vi "10-send&receive-arrays-backup2.vi"() -> ()   [LabVIEW 2018]
uses:
  LV2Julia_core/VIs/Server or client state.ctl
  LV2Julia_core/VIs/detailed error info.ctl
  LV2Julia_core/VIs/StackFrame.ctl
  LV2Julia_core/VIs/Numeric Types enum.ctl
  array 123D sizes.ctl
  LV2Julia_core/VIs/Commands.ctl
  19565153-6e23-41a7-814d-e58de81dde5a.vi
  5ef99b4f-9bfc-4a0d-a8a0-74b261859f3d.vi
  388a3b2a-e541-4e37-ba3b-5749cefc77c1.vi
  e91abbe1-2489-4f0d-9743-379a6a4cbf4d.vi
  19565153-6e23-41a7-814d-e58de81dde5a.vi/85887d54-d509-450b-84bb-3c420582994f.vi
  <vilib>/Utility/High Resolution Relative Seconds.vi
  388a3b2a-e541-4e37-ba3b-5749cefc77c1.vi/1b30b06e-7fd1-4fdb-a624-ecc8bbac65c1.vi
  19565153-6e23-41a7-814d-e58de81dde5a.vi/85887d54-d509-450b-84bb-3c420582994f.vi/d3e8bd18-7aca-49eb-9cc1-8936944af3d1.vi
  19565153-6e23-41a7-814d-e58de81dde5a.vi/85887d54-d509-450b-84bb-3c420582994f.vi/cc0638ed-03b9-4f11-90bc-5f951413100e.vi
  19565153-6e23-41a7-814d-e58de81dde5a.vi/85887d54-d509-450b-84bb-3c420582994f.vi/437cd6de-f34e-42af-877a-dd33a1fabbe3.vi
  388a3b2a-e541-4e37-ba3b-5749cefc77c1.vi/1b30b06e-7fd1-4fdb-a624-ecc8bbac65c1.vi/cb39e787-6450-4332-a618-a02e848b2eda.vi
  388a3b2a-e541-4e37-ba3b-5749cefc77c1.vi/1b30b06e-7fd1-4fdb-a624-ecc8bbac65c1.vi/8ffec59d-6774-4d31-b6e2-7d50134dbb1f.vi
  388a3b2a-e541-4e37-ba3b-5749cefc77c1.vi/1b30b06e-7fd1-4fdb-a624-ecc8bbac65c1.vi/38fcd616-394b-4d55-b8d7-64853e38e30b.vi
  LV2Julia_core/VIs/jl-scripts path.vi
  LV2Julia_core/VIs/check ID validity.vi
  LV2Julia_core/VIs/bindata_descr to JSON.vi
  LV2Julia_core/VIs/check cluster field names.vi
  LV2Julia_core/VIs/concat JSON.vi
  LV2Julia_core/VIs/build request.vi
  LV2Julia_core/VIs/Parse server response.vi
  LV2Julia_core/VIs/log jl exceptions.vi
  LV2Julia_core/LV2Julia_core.lvlib
  LV2Julia_examples.lvlib
panel:
  out "ZMQ timeout":bool
  out "Julia script file path":path
  out "temporary script path":path
  in  "execution control pages":enum32{"Start&stop", "go - test", "error"}(tab)
  in  "returnarrs":bool=TRUE
  in  "go":bool caption="go (Julia Server started externally)"
  in  "Start with Julia":bool caption="Start Julia Server and go"
  in  "ZMQ endpoint":string="tcp://127.0.0.1:5555"
  out "Jl Server state":T1
  in  "stop this VI only":bool
  in  "stop both this VI and Julia Server":bool
  in  "Stop JL-server":bool
  in  "log2(arrsize)":u32=7 min=5
  in  "cycle min time (s)":sgl min=0 step=0.2
  out "numarray 3D":cdb[][][](array[numeric])
  out "numarray 2D":cdb[][](array[numeric])
  out "numarray 1D":cdb[](array[numeric]) format="%.1f"
  out "numeric type":T2
  out "arr dimension":i32
  out "all arrays OK":bool
  out "arrs equal":bool
  out "array sizes":T3
  out "el_type":string
  out "arsize":i32[](array[numeric])
  out "data flattening delta t":dbl
  out "flattening ms/MB":dbl format="%#.2f"
  out "Zmq&Julia delta t":dbl
  out "Zmq&JUlia ms/MB":dbl format="%#.2f"
  out "data unflattening delta t":dbl
  out "unflattening ms/MB":dbl format="%#.2f"
  out "detailed error info":T4
  out "current error":errorcluster
  out "final error":errorcluster
  out "short err code":u8
  # "tcp://127.0.0.1:5555 \nfor local Julia Server\n\nFor a Julia Server running on a separate computer,  you probably must use an IPv4 address in numeric form (not a DNS name) - see https://stackoverflow.com/questions/6024003/why-doesnt-zeromq-work-on-localhost.\n\nFor instructions how to properly start the corresponding Julia script, see \n05-on_external_server.jl file in the jl-scripts folder.\n\nThe ZMQ endpoint control only used if Julia Server is not being started by this VI."
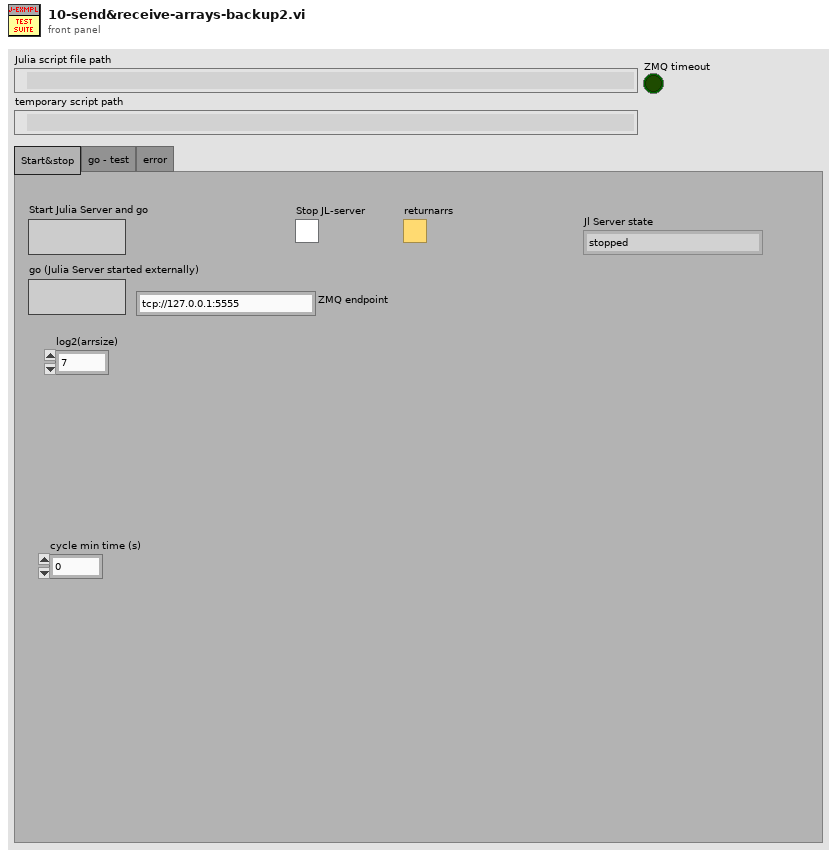
[diagram p1: front panel]
types:
  T1 = typedef "LV2Julia_core.lvlib/Server or client state.ctl" = enum16{"stopped", "running", "unknown"}
  T2 = typedef "LV2Julia_core.lvlib/Numeric Types enum.ctl" = enum16{"SGL", "DBL", "I8", "I16", "I32", "I64", "U8", "U16", "U32", "U64", "CSGL", "CDBL", "boolean"}
  T3 = typedef "array 123D sizes.ctl" = cluster{"s1":i32, "s2":i32[], "s3":i32[]}
  T4 = typedef "LV2Julia_core.lvlib/detailed error info.ctl" = cluster{"exception_or_info":string, "trace":T5[]}
  T5 = typedef "LV2Julia_core.lvlib/StackFrame.ctl" = cluster{"frame_summary":string, "func":string, "linfo":string, "file":string, "line":i32, "pointer":u64, "from_c":bool, "inlined":bool}
  T6 = typedef "LV2Julia_core.lvlib/Commands.ctl" = enum16{"Start Jl-server & Init LV-client", "Send request & Get response ", "Stop Jl-server & Cleanup LV-client", "Cleanup LV-client", "Start Jl-server", "Stop Jl-server", "Init LV-Client", "Cleanup LV-Client", "(not allowed)", "Set LV Client state", "Set Jl Server state", "set ZMQ timeout", "read ZMQ timeout", "read-out state"}
  T7 = typedef "LV2Julia_core.lvlib/Bindata&description.ctl" = cluster{"bindata_descr":T8[], "bindata":u8[]}
  T8 = typedef "LV2Julia_core.lvlib/Bindata description.ctl" = cluster{"nofbytes":i32, "numtype":string, "start":i32, "arrdims":i32[], "kwarg_name":string, "category":string}
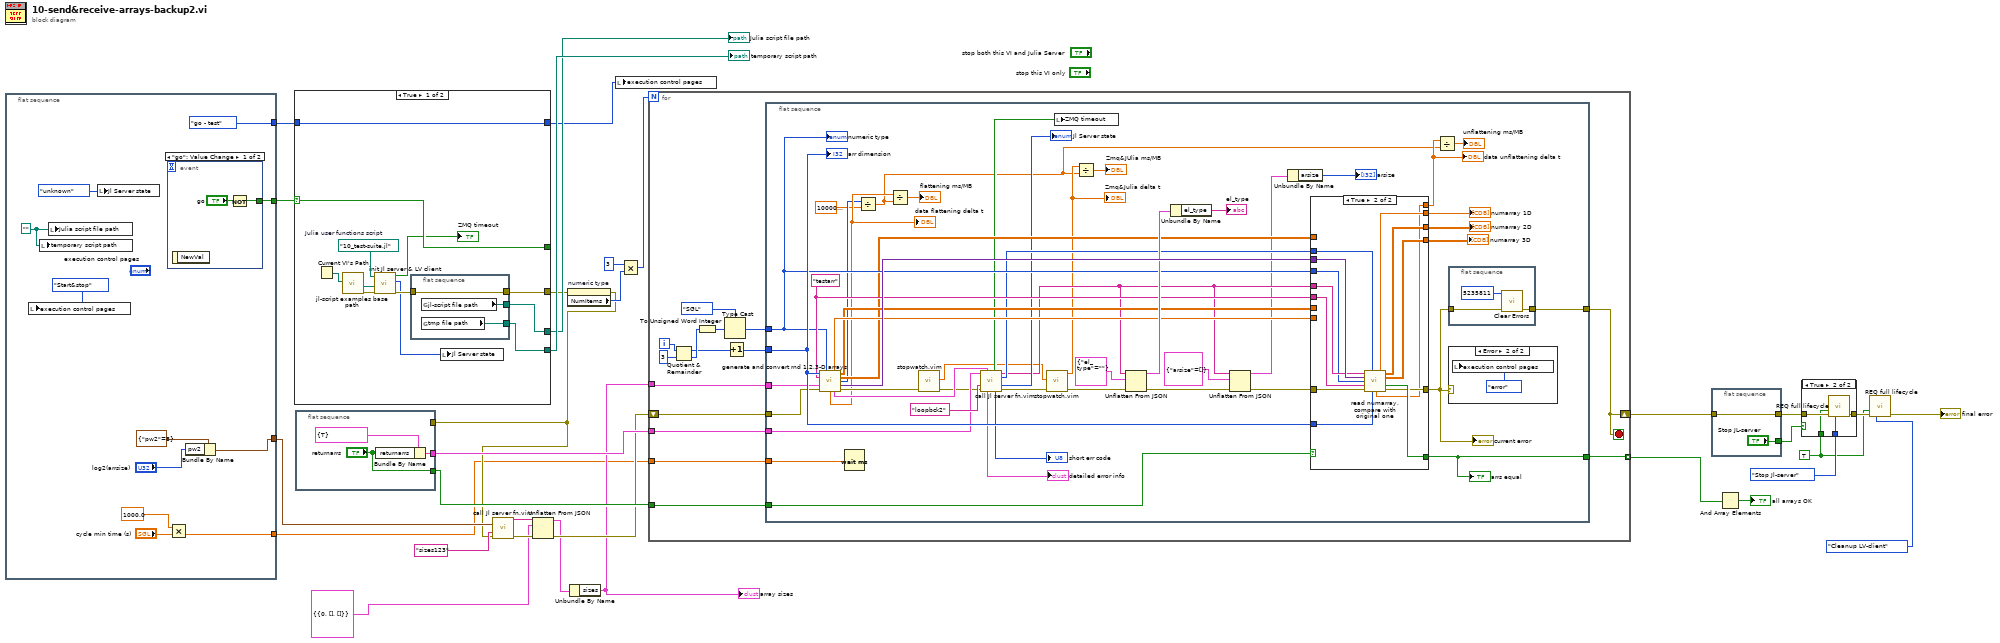
[diagram p0: block diagram]
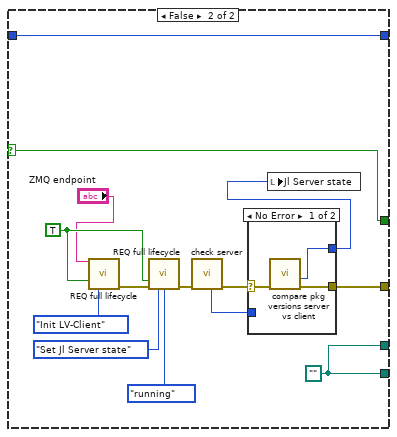
[diagram p2: hidden frame]
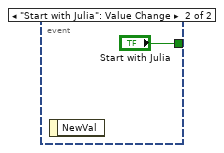
[diagram p4: hidden frame]
diagram:
  w27 = TRUE ("Force command")
  n1 = flat-sequence {
    tunnel: [w40] -> w20
    tunnel: [enum32{"Start&stop", "go - test", "error"}."go - test" ("execution control pages")] -> w15
    tunnel: [w36] -> w9
    tunnel: [w33] -> w1
    frame #0 {
      w41 = path ""
      n2 = local write "execution control pages"(enum32{"Start&stop", "go - test", "error"}."Start&stop" ("execution control pages")) -> ()
      n3 = local write "temporary script path"(w41) -> ()
      n4 = local write "Julia script file path"(w41) -> ()
      n5 = local write "Jl Server state"(Server_or_client_state."unknown" ("Jl Server state out")) -> ()
      n6 = event shown="[0] \"go\": Value Change" {
        selector: _ -> [_ _]
        dyn-events: _ -> [_ _]
        timeout: _ -> [_ _]
        tunnel: [w43 "Start with Julia"] -> w40
        event "go": Value Change {
          n7 = event-data() -> ()  [unwired: 1 in, 1 out]
          n8 = Not(x="go") -> (.not. x?=w43:bool)
        }
        event "Start with Julia": Value Change {
          n9 = event-data() -> ()  [unwired: 1 in, 1 out]
        }
      }
      n10 = Multiply(x=sgl 1000.0, y="cycle min time (s)") -> (x*y=w33:sgl)
      n11 = Bundle By Name(cluster=cluster{"pw2":u32} {"pw2"=8}, "pw2"="log2(arrsize)") -> (w36:cluster{"pw2":u32})
    }
  }
  n12 = case shown="True" w20 {
    selector: w20 -> [w57 w70]
    tunnel: [w56 w65] -> w17
    tunnel: [w57 w70] -> _
    tunnel: [w55 w67] -> w18
    tunnel: [w54 w67] -> w19
    tunnel: [w46 w61] -> w16
    tunnel: w15 -> [w46 w61]
    frame True {
      w48 = path "10_test-suite.jl"  # Julia user functions script
      n13 = Current VI's Path() -> (path=w52:path)
      n14 = call "jl-script examples base path.vi"("calling example VI path"=w52) -> ("error out"=w51:errorcluster, "jl-script-examples base path"=w50:path)  [unwired: 9 in]
      n15 = call "init Jl server & LV client.vi"("error in (no error)"=w51, "Base path (not a path)"=w50, "Julia user functions script"=w48) -> ("error out"=w53:errorcluster, "Jl Server state out"=w49:T1, "timeout?"=→"ZMQ timeout":bool)  [unwired: 6 in]
      n16 = flat-sequence {
        tunnel: [w60] -> w56
        tunnel: w53 -> [w60]
        tunnel: [w59] -> w55
        tunnel: [w58] -> w54
        frame #0 {
          n17 = global read "jl-scripts path.vi" "jl-script file path"() -> (w59:path)
          n18 = global read "jl-scripts path.vi" "tmp file path"() -> (w58:path)
        }
      }
      n19 = local write "Jl Server state"(w49) -> ()
    }
    frame False {
      w67 = path ""
      w72 = TRUE ("Force command")
      n20 = call "REQ full lifecycle.vi"("ZMQ endpoint"="ZMQ endpoint", "Force command"=w72, "command"=Commands."Init LV-Client") -> ("error out"=w69:errorcluster)  [unwired: 6 in, 6 out]
      n21 = call "REQ full lifecycle.vi"("Force command"=w72, "error in"=w69, "command"=Commands."Set Jl Server state", "Jl Server state in"=Server_or_client_state."running") -> ("error out"=w68:errorcluster)  [unwired: 5 in, 6 out]
      n22 = call "check server.vi"("error in"=w68) -> ("error out"=w66:errorcluster, "Jl Server state out"=w64:T1)  [unwired: 6 in, 3 out]
      n23 = case shown="No Error" w66 {
        selector: w66 -> [w77 w79]
        tunnel: [w76 w79] -> w65
        tunnel: [w75 w78] -> w62
        tunnel: w64 -> [_ w78]
        frame No Error {
          n24 = call "compare pkg versions server vs client.vi"("error in (no error)"=w77) -> ("error out"=w76:errorcluster, "Jl Server state out"=w75:T1)  [unwired: 4 in, 5 out]
        }
        frame Error {
        }
      }
      n25 = local write "Jl Server state"(w62) -> ()
    }
  }
  "temporary script path" <- w19
  "Julia script file path" <- w18
  n26 = flat-sequence {
    tunnel: [w81] -> w14
    tunnel: ["returnarrs"] -> w13
    tunnel: w8 -> [_]
    frame #0 {
      n27 = Bundle By Name(cluster=cluster{"returnarrs":bool} {"returnarrs"=TRUE}, "returnarrs"="returnarrs") -> (w81:cluster{"returnarrs":bool})
    }
  }
  n28 = property on="numeric type" class="Enum (strict)"(error in=w17) -> (error out=w8:errorcluster, "NumItems"=w25:u32)  [unwired: 1 in, 1 out]
  n29 = call "call Jl server fn.vim"("Arguments 2"=w9, "fun2call"="sizes123", "error in (no error)"=w8) -> ("JSON received"=w5:string, "error out"=w7:errorcluster)  [unwired: 6 in, 5 out]
  n30 = Unflatten From JSON(JSON string=w5, type and defaults=cluster{"sizes":T3} {"sizes"={"s1"=0, "s2"=[], "s3"=[]}}, error in (no error)=w7) -> (value=w4:cluster{"sizes":T3}, error out=w6:errorcluster)  [unwired: 4 in]
  n31 = Unbundle By Name(w4) -> ("sizes"=w2:T3)
  "array sizes" <- w2
  n32 = local write "execution control pages"(w16) -> ()
  n33 = Multiply(x=u32 3, y=w25) -> (x*y=w23:u32)
  n34 = for {
    N: w23 -> [_]
    tunnel: [w83] -> w22 mode=indexing
    shift-right: [w89] -> w12
    shift-left: w6 -> [w90]
    tunnel: w14 -> [w86]
    tunnel: w13 -> [w87]
    tunnel: w2 -> [w85]
    tunnel: w1 -> [w84]
    i -> [w97]
    stop <- w89 stop-if-true
    n35 = Quotient & Remainder(x=w97, y=3) -> (x-y*floor(x/y)=w92:i32, floor(x/y)=w93:i32)
    n36 = To Unsigned Word Integer(number=w93) -> (unsigned 16bit integer=w94:u16)
    n37 = Type Cast(type=Numeric_Types_enum."SGL" ("numeric type const"), x=w94) -> (*(type *) &x=w88:T2)
    n38 = Increment(x=w92) -> (x+1=w91:i32)
    n39 = flat-sequence {
      tunnel: w91 -> [w142]
      tunnel: w90 -> [w141]
      tunnel: [w140] -> w89
      tunnel: w88 -> [w135]
      tunnel: w87 -> [w132]
      tunnel: w86 -> [w127]
      tunnel: w85 -> [w120]
      tunnel: w84 -> [w119]
      tunnel: [w100] -> w83
      frame #0 {
        w136 = "testarr" ("Tag")
        n40 = call "generate and convert rnd 1,2,3-D arrays.vi"("dims"=w142, "numeric type const"=w135, "Tag"=w136, "sizes"=w120, "error in (no error)"=w141) -> ("Array 1D"=w131:cdb[], "Array 2D"=w130:cdb[][], "Array 3D"=w129:cdb[][][], "bytes"=w101:i32, "array as variant"=w144:variant, "delta t (s)"=w107:dbl, "Bindata & descr out"=w122:T7, "error out"=w111:errorcluster)  [unwired: 1 in, 2 out]
        "data flattening delta t" <- w107
        n41 = Wait (ms)(milliseconds to wait=w119) -> ()  [unwired: 1 out]
        n42 = Divide(x=w101, y=1000000000.0) -> (x/y=w98:dbl)
        n43 = Divide(x=w107, y=w98) -> (x/y=→"flattening ms/MB":dbl)
        n44 = call "stopwatch.vim"("anything in"=w111) -> ("copy of anything out"=w110:errorcluster, "current timepoint"=w112:dbl)  [unwired: 8 in, 1 out]
        n45 = call "call Jl server fn.vim"("Arguments 1"=w127, "Bindata & descr in"=w122, "fun2call"="loopbck2", "error in (no error)"=w110) -> ("timeout?"=w121:bool, "JSON received"=w116:string, "binary data received"=w125:u8[], "Jl Server state out"=→"Jl Server state":T1, "detailed error info"=→"detailed error info":T4, "return code"=→"short err code":u8, "error out"=w109:errorcluster)  [unwired: 5 in]
        n46 = call "stopwatch.vim"("anything in"=w109, "prev timepoint (0)"=w112) -> ("copy of anything out"=w108:errorcluster, "delta t (s)"=w104:dbl)  [unwired: 7 in, 1 out]
        "Zmq&Julia delta t" <- w104
        n47 = local write "ZMQ timeout"(w121) -> ()
        n48 = Divide(x=w104, y=w98) -> (x/y=→"Zmq&JUlia ms/MB":dbl)
        n49 = Unflatten From JSON(JSON string=w116, type and defaults=cluster{"el_type":string} {"el_type"=""} ("parsed response"), error in (no error)=w108) -> (value=w139:cluster{"el_type":string}, error out=w118:errorcluster)  [unwired: 4 in]
        n50 = Unbundle By Name(w139) -> ("el_type"=→"el_type":string)
        n51 = Unflatten From JSON(JSON string=w116, type and defaults=cluster{"arsize":i32[]} {"arsize"=[]} ("parsed response"), error in (no error)=w118) -> (value=w114:cluster{"arsize":i32[]}, error out=w117:errorcluster)  [unwired: 4 in]
        n52 = Unbundle By Name(w114) -> ("arsize"=→"arsize":i32[])
        n53 = case shown="True" w132 {
          tunnel: w125 -> [_ w162]
          tunnel: [w148 w161] -> w145
          tunnel: w144 -> [_ w160]
          tunnel: [w146 w159] -> w143
          tunnel: [_ w158] -> w100
          tunnel: w142 -> [_ w157]
          tunnel: w117 -> [w149 w156]
          tunnel: w116 -> [_ w155]
          tunnel: w136 -> [_ w154]
          tunnel: w135 -> [_ w153]
          tunnel: [w147 w152] -> w134
          tunnel: [w149 w151] -> w133
          tunnel: w131 -> [w148 _]
          tunnel: w130 -> [w147 _]
          tunnel: w129 -> [w146 _]
          tunnel: [_ w150] -> w102
          frame False {
          }
          frame True {
            n54 = call "read numarray, compare with original one.vi"("JSON in"=w155, "binary data in"=w162, "array as variant in"=w160, "numeric type"=w153, "kwarg_name"=w154, "error in (no error)"=w156, "dims"=w157) -> ("numarray 1D"=w161:cdb[], "numarray 2D"=w152:cdb[][], "numarray 3D"=w159:cdb[][][], "arrays are equal"=w158:bool, "delta t (s)"=w150:dbl, "error out"=w151:errorcluster)  [unwired: 1 in, 2 out]
          }
        }
        "numarray 1D" <- w145
        "arrs equal" <- w100
        "numarray 2D" <- w134
        "numarray 3D" <- w143
        "current error" <- w133
        "data unflattening delta t" <- w102
        n55 = Divide(x=w102, y=w98) -> (x/y=→"unflattening ms/MB":dbl)
        n56 = flat-sequence {
          tunnel: w133 -> [w166]
          tunnel: [w165] -> w140
          frame #0 {
            n57 = call <vilib>:"Clear Errors.vi"("error in (no error)"=w166, "specific error code to clear (0: all)"=5235811) -> ("error out"=w165:errorcluster)  [unwired: 4 in, 1 out]
          }
        }
        n58 = case shown="Error" w133 {
          frame No Error {
          }
          frame Error {
            n59 = local write "execution control pages"(enum32{"Start&stop", "go - test", "error"}."error" ("execution control pages")) -> ()
          }
        }
        "numeric type" <- w135
        "arr dimension" <- w142
      }
    }
  }
  n60 = flat-sequence {
    tunnel: ["Stop JL-server"] -> w26
    tunnel: [w167] -> w11
    tunnel: w12 -> [w167]
    frame #0 {
    }
  }
  n61 = And Array Elements(Boolean array=w22) -> (logical AND=→"all arrays OK":bool)
  n62 = case shown="True" w26 {
    tunnel: w11 -> [w169 w173]
    tunnel: Commands."Stop Jl-server" ("command") -> [_ w172]
    tunnel: [w169 w171] -> w30
    tunnel: w27 -> [_ w170]
    frame False {
    }
    frame True {
      n63 = call "REQ full lifecycle.vi"("Force command"=w170, "error in"=w173, "command"=w172) -> ("error out"=w171:errorcluster)  [unwired: 6 in, 6 out]
    }
  }
  n64 = call "REQ full lifecycle.vi"("Force command"=w27, "error in"=w30, "command"=Commands."Cleanup LV-client") -> ("error out"=→"final error":errorcluster)  [unwired: 6 in, 6 out]
